vi "Baxter.vi"() -> ()   [LabVIEW 2010]
panel:
  out "sdf out":string
  out "3D Picture":refnum<vi>(3d-picture)
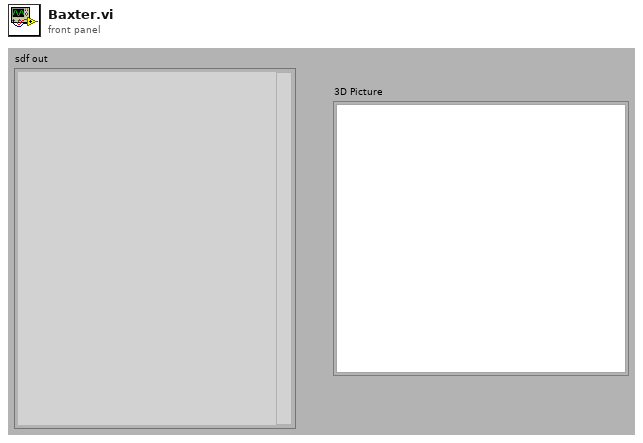
[diagram p1: front panel]
types:
  T1 = cluster{"X":sgl, "Y":sgl, "Z":sgl, "roll":sgl, "pitch":sgl, "yaw":sgl}
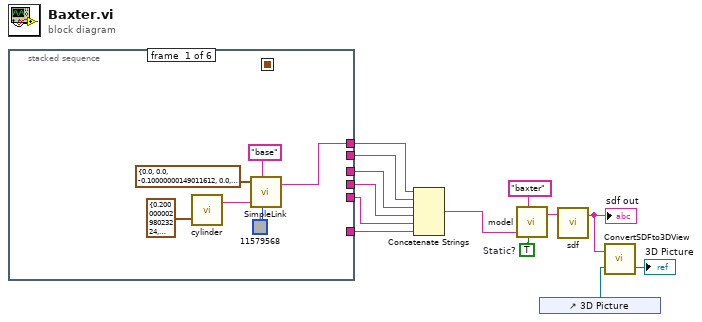
[diagram p0: block diagram]
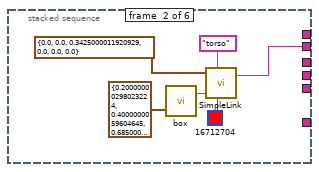
[diagram p2: hidden frame]
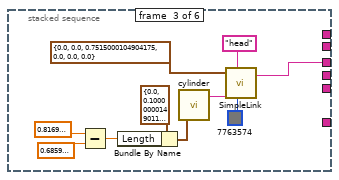
[diagram p3: hidden frame]
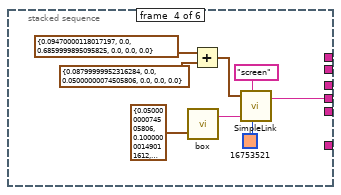
[diagram p4: hidden frame]
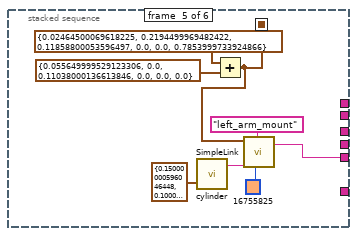
[diagram p5: hidden frame]
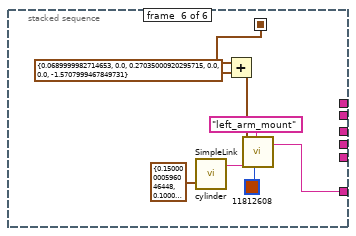
[diagram p6: hidden frame]
diagram:
  w10 = TRUE  # Static?
  n1 = stacked-sequence {
    seq-local: [_ _ _ _ w44 _] -> [_ _ _ _ _ w53]
    tunnel: [w14 _ _ _ _ _] -> w7
    tunnel: [_ w20 _ _ _ _] -> w6
    tunnel: [_ _ w32 _ _ _] -> w5
    tunnel: [_ _ _ w39 _ _] -> w4
    tunnel: [_ _ _ _ w47 _] -> w3
    tunnel: [_ _ _ _ _ w52] -> w2
    frame #0 {
      n2 = call "cylinder.vi"("Cylinder"=cluster{"Length":sgl, "Radius":sgl} {"Length"=0.2, "Radius"=0.1}) -> ("urdf out"=w18:string)  [unwired: 3 in]
      n3 = call "SimpleLink.vi"("Geometry"=T1 {"X"=0.0, "Y"=0.0, "Z"=-0.1, "roll"=0.0, "pitch"=0.0, "yaw"=0.0} ("Pose"), "Name"="base", "mass"=w18, "link color"=u32 11579568) -> ("link out"=w14:string)  [unwired: 2 in]
    }
    frame #1 {
      n4 = call "box.vi"("Box"=cluster{"Length":sgl, "Width":sgl, "Height":sgl} {"Length"=0.2, "Width"=0.4, "Height"=0.685}) -> ("urdf out"=w23:string)  [unwired: 3 in]
      n5 = call "SimpleLink.vi"("Geometry"=T1 {"X"=0.0, "Y"=0.0, "Z"=0.3425, "roll"=0.0, "pitch"=0.0, "yaw"=0.0} ("Pose"), "Name"="torso", "mass"=w23, "link color"=u32 16712704) -> ("link out"=w20:string)  [unwired: 2 in]
    }
    frame #2 {
      n6 = Subtract(x=sgl 0.817 ("Z"), y=sgl 0.686 ("Z")) -> (x-y=w26:sgl)
      n7 = Bundle By Name(cluster=cluster{"Length":sgl, "Radius":sgl} {"Length"=0.0, "Radius"=0.1} ("Cylinder"), "Length"=w26) -> (w27:cluster{"Length":sgl, "Radius":sgl})
      n8 = call "cylinder.vi"("Cylinder"=w27) -> ("urdf out"=w31:string)  [unwired: 3 in]
      n9 = call "SimpleLink.vi"("Geometry"=T1 {"X"=0.0, "Y"=0.0, "Z"=0.7515, "roll"=0.0, "pitch"=0.0, "yaw"=0.0} ("Pose"), "Name"="head", "mass"=w31, "link color"=u32 7763574) -> ("link out"=w32:string)  [unwired: 2 in]
    }
    frame #3 {
      n10 = call "box.vi"("Box"=cluster{"Length":sgl, "Width":sgl, "Height":sgl} {"Length"=0.05, "Width"=0.1, "Height"=0.1}) -> ("urdf out"=w41:string)  [unwired: 3 in]
      n11 = Add(x=T1 {"X"=0.0947, "Y"=0.0, "Z"=0.686, "roll"=0.0, "pitch"=0.0, "yaw"=0.0} ("Pose"), y=T1 {"X"=0.088, "Y"=0.0, "Z"=0.05, "roll"=0.0, "pitch"=0.0, "yaw"=0.0} ("Pose")) -> (x+y=w36:T1)
      n12 = call "SimpleLink.vi"("Geometry"=w36, "Name"="screen", "mass"=w41, "link color"=u32 16753521) -> ("link out"=w39:string)  [unwired: 2 in]
    }
    frame #4 {
      n13 = call "cylinder.vi"("Cylinder"=cluster{"Length":sgl, "Radius":sgl} {"Length"=0.15, "Radius"=0.1}) -> ("urdf out"=w48:string)  [unwired: 3 in]
      n14 = Add(x=T1 {"X"=0.024645, "Y"=0.21945, "Z"=0.118588, "roll"=0.0, "pitch"=0.0, "yaw"=0.7854} ("Pose"), y=T1 {"X"=0.05565, "Y"=0.0, "Z"=0.11038, "roll"=0.0, "pitch"=0.0, "yaw"=0.0} ("Pose")) -> (x+y=w44:T1)
      n15 = call "SimpleLink.vi"("Geometry"=w44, "Name"="left_arm_mount", "mass"=w48, "link color"=u32 16755825) -> ("link out"=w47:string)  [unwired: 2 in]
    }
    frame #5 {
      n16 = call "cylinder.vi"("Cylinder"=cluster{"Length":sgl, "Radius":sgl} {"Length"=0.15, "Radius"=0.1}) -> ("urdf out"=w56:string)  [unwired: 3 in]
      n17 = Add(x=w53, y=T1 {"X"=0.069, "Y"=0.0, "Z"=0.27035, "roll"=0.0, "pitch"=0.0, "yaw"=-1.5708} ("Pose")) -> (x+y=w54:T1)
      n18 = call "SimpleLink.vi"("Geometry"=w54, "Name"="left_arm_mount", "mass"=w56, "link color"=u32 11812608) -> ("link out"=w52:string)  [unwired: 2 in]
    }
  }
  n19 = Concatenate Strings(w7, w6, w5, w4, w3, w2) -> (w8:string)
  n20 = call "model.vi"("Name"="baxter", "joints"=w8, 4:w10) -> ("urdf out"=w11:string)  [unwired: 3 in]
  n21 = control-ref of="3D Picture"() -> (w1:refnum<vi>)
  n22 = call "sdf.vi"("assets"=w11) -> ("sdf out"=w12:string)  [unwired: 2 in]
  "sdf out" <- w12
  n23 = call "ConvertSDFto3DView.vi"("SceneGraphDisp Refnum"=w1, "urdf"=w12) -> ("3D Picture"=→"3D Picture":refnum<vi>)  [unwired: 1 out]
